vi "Read Play sound when done.vi"(11 "Test Framework in":refnum<class "Test Framework.lvclass">) -> (2 "Play sound when done":bool, 3 "Test Framework out":refnum<class "Test Framework.lvclass">)   [LabVIEW 2020, in "Test Framework.lvclass"]
uses:
  Test Framework.lvclass
  Test Framework.lvclass/Test Framework.ctl
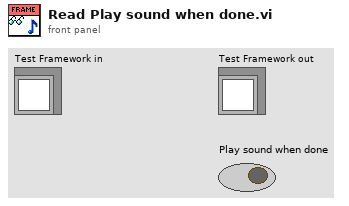
[diagram p1: front panel]
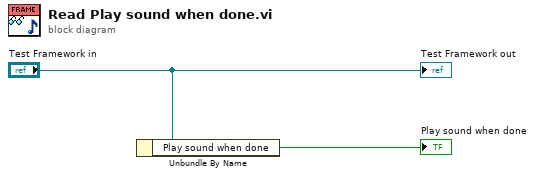
[diagram p0: block diagram]
diagram:
  n1 = Unbundle By Name("Test Framework in") -> ("Play sound when done"=→"Play sound when done":bool)
  "Test Framework out" <- "Test Framework in"
